vi "regUserEvent.vi"(8 "error in (no error)":errorcluster, 11 "tcpServerCmd in":refnum<class "TcpServerCmd.lvclass">) -> (0 "error out":errorcluster, 3 "tcpServerCmd out":refnum<class "TcpServerCmd.lvclass">)   [LabVIEW 2018, in "TcpServerCmd.lvclass"]
doc: "Register User Events."
uses:
  TcpServerCmd.lvclass
  typedef/ackTypeDef.ctl
  typedef/userEventTypeDef.ctl
  typedef/eventTypeDef.ctl
  TcpServerCmd.lvclass/TcpServerCmd.ctl
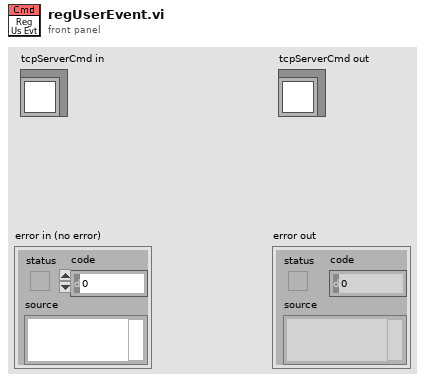
[diagram p1: front panel]
types:
  T1 = typedef "TcpServerCmd.lvclass/userEventTypeDef.ctl" = cluster{"CmdRead":refnum<user-event>, "CmdWrite":refnum<user-event>, "EvtRead":refnum<user-event>, "EvtWrite":refnum<user-event>, "GenRead":refnum<user-event>, "GenWrite":refnum<user-event>}
  T2 = typedef "TcpServerCmd.lvclass/eventTypeDef.ctl" = cluster{"name":string, "evtlDetails":string}
  T3 = typedef "TcpServerCmd.lvclass/ackTypeDef.ctl" = cluster{"packet":string, "cmdStatus":string}
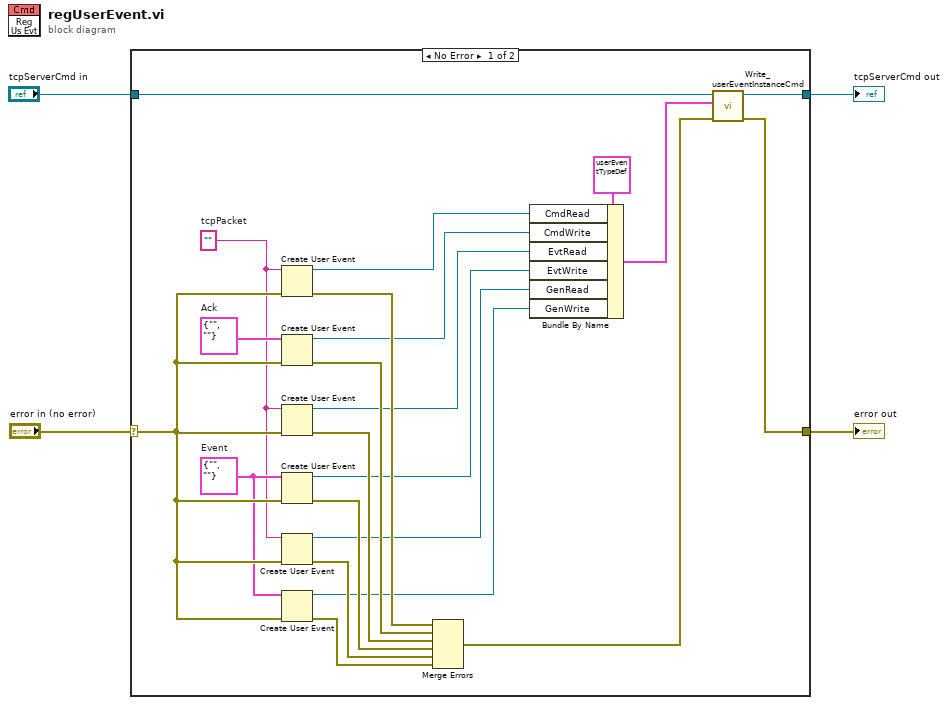
[diagram p0: block diagram]
diagram:
  n1 = case shown="No Error" "error in (no error)" {
    selector: "error in (no error)" -> [w13 w28]
    tunnel: [w24 w28] -> w3
    tunnel: [w25 w27] -> w1
    tunnel: "tcpServerCmd in" -> [w26 w27]
    frame No Error {
      w5 = ""  # tcpPacket
      w10 = T2 {"name"="", "evtlDetails"=""}  # Event
      w22 = T3 {"packet"="", "cmdStatus"=""}  # Ack
      n2 = Create User Event(user event datatype=w5, error in=w13) -> (user event=w16:refnum<user-event>, error out=w20:errorcluster)
      n3 = Create User Event(user event datatype=w22, error in=w13) -> (user event=w15:refnum<user-event>, error out=w19:errorcluster)
      n4 = Create User Event(user event datatype=w5, error in=w13) -> (user event=w7:refnum<user-event>, error out=w18:errorcluster)
      n5 = Create User Event(user event datatype=w10, error in=w13) -> (user event=w9:refnum<user-event>, error out=w14:errorcluster)
      n6 = Create User Event(user event datatype=w5, error in=w13) -> (user event=w6:refnum<user-event>, error out=w12:errorcluster)
      n7 = Create User Event(user event datatype=w10, error in=w13) -> (user event=w8:refnum<user-event>, error out=w11:errorcluster)
      n8 = Merge Errors(w20, w19, w18, w14, w12, w11) -> (w21:errorcluster)
      n9 = Bundle By Name(cluster=T1 {"CmdRead"=refnum, "CmdWrite"=refnum, "EvtRead"=refnum, "EvtWrite"=refnum, "GenRead"=refnum, "GenWrite"=refnum} ("userEventInstancesCmd"), "CmdRead"=w16, "CmdWrite"=w15, "EvtRead"=w7, "EvtWrite"=w9, "GenRead"=w6, "GenWrite"=w8) -> (w23:T1)
      n10 = call "Write_userEventInstanceCmd.vi"("error in (no error)"=w21, "userEventInstanceCmd"=w23, "TcpServerCmd in"=w26) -> ("error out"=w24:errorcluster, "TcpServerCmd out"=w25:refnum<class "TcpServerCmd.lvclass">)  [unwired: 7 in]
    }
    frame Error {
    }
  }
  "error out" <- w3
  "tcpServerCmd out" <- w1
